vi "Correct_Position_info.vi"() -> (0 "error out":errorcluster, 4 "Path":path)   [LabVIEW 2015]
panel:
  out "File Changed":bool
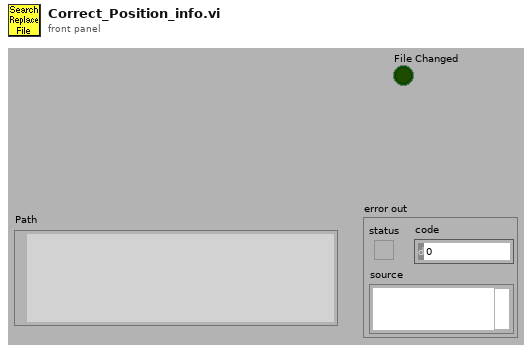
[diagram p1: front panel]
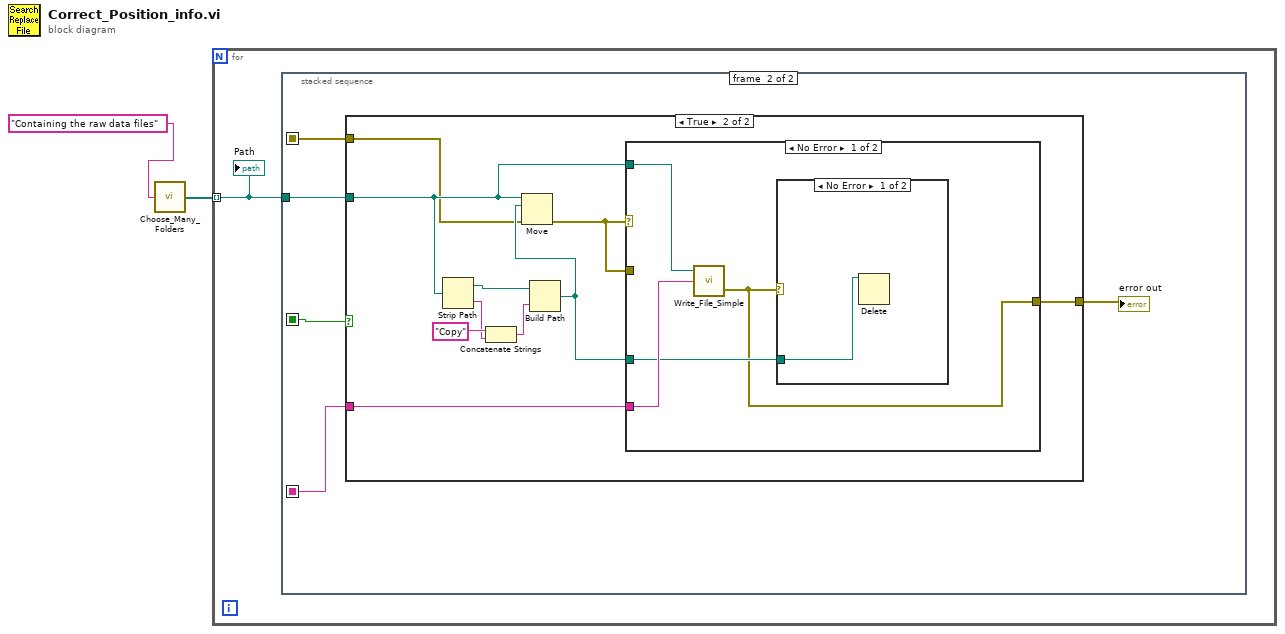
[diagram p0: block diagram]
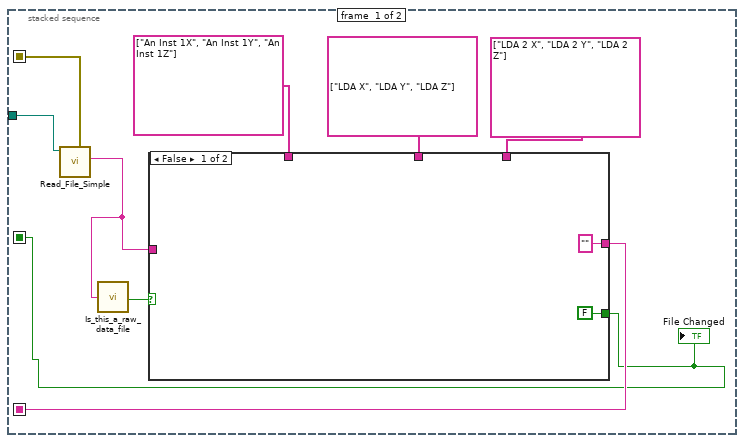
[diagram p2: hidden frame]
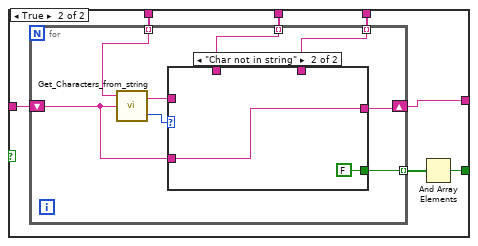
[diagram p3: hidden frame]
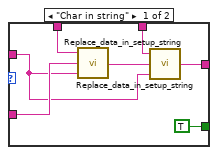
[diagram p4: hidden frame]
diagram:
  n1 = call "Choose_Many_Folders.vi"("Purpose of choosing folder"="Containing the raw data files") -> ("Files"=w1:path[])
  n2 = for {
    tunnel: w1 -> [w3] mode=indexing
    n3 = stacked-sequence {
      seq-local: [w11 _] -> [_ w39]
      seq-local: [w8 _] -> [_ w41]
      seq-local: [w6 _] -> [_ w40]
      tunnel: w3 -> [w12 w43]
      frame #0 {
        n4 = call "Read_File_Simple.vi"("Filename"=w12) -> ("error out"=w11:errorcluster, "string"=w5:string)  [unwired: 4 in, 4 out]
        n5 = call "Is_this_a_raw_data_file.vi"("character string"=w5) -> ("Raw Dat File?"=w4:bool)  [unwired: 2 out]
        n6 = case shown="False" w4 {
          tunnel: string[] ["An Inst 1X", "An Inst 1Y", "An Inst 1Z"] -> [_ w21]
          tunnel: string[] ["LDA X", "LDA Y", "LDA Z"] -> [_ w20]
          tunnel: ["" ("string") w19] -> w8
          tunnel: string[] ["LDA 2 X", "LDA 2 Y", "LDA 2 Z"] -> [_ w18]
          tunnel: [FALSE w16] -> w6
          tunnel: w5 -> [_ w15]
          frame False {
          }
          frame True {
            n7 = for {
              shift-right: [w25] -> w19
              shift-left: w15 -> [w26]
              tunnel: w21 -> [w29] mode=indexing
              tunnel: w20 -> [w28] mode=indexing
              tunnel: w18 -> [w27] mode=indexing
              tunnel: [w22] -> w17 mode=indexing
              n8 = call "Get_Characters_from_string.vi"("Input string"=w26, "Variable name"=w29) -> ("Status"=w23:enum16{"Char in string", "Char not in string"}, "Value"=w24:string)  [unwired: 1 in]
              n9 = case shown="\"Char not in string\"" w23 {
                tunnel: w28 -> [w36 _]
                tunnel: w27 -> [w35 _]
                tunnel: w26 -> [w34 w38]
                tunnel: [w33 w38] -> w25
                tunnel: w24 -> [w31 _]
                tunnel: [TRUE FALSE] -> w22
                frame "Char in string" {
                  n10 = call "Replace_data_in_setup_string.vi"("New data string"=w31, "Input string"=w34, "Variable name"=w36) -> ("Appended string"=w32:string)
                  n11 = call "Replace_data_in_setup_string.vi"("New data string"=w31, "Input string"=w32, "Variable name"=w35) -> ("Appended string"=w33:string)
                }
                frame "Char not in string" {
                }
              }
            }
            n12 = And Array Elements(Boolean array=w17) -> (logical AND=w16:bool)
          }
        }
        "File Changed" <- w6
      }
      frame #1 {
        n13 = case shown="True" w40 {
          tunnel: w43 -> [_ w50]
          tunnel: w41 -> [_ w49]
          tunnel: [w44 w47] -> w42
          tunnel: w39 -> [w44 w45]
          frame False {
          }
          frame True {
            n14 = Strip Path(path=w50) -> (stripped path=w51:path, name=w53:string)
            n15 = Concatenate Strings("Copy" ("name or relative path"), w53) -> (w52:string)
            n16 = Build Path(base path=w51, name or relative path=w52) -> (appended path=w48:path)
            n17 = Move(source path=w50, error in=w45, 10:w48) -> (error out=w46:errorcluster)  [unwired: 2 in, 2 out]
            n18 = case shown="No Error" w46 {
              tunnel: w50 -> [w58 _]
              tunnel: w49 -> [w57 _]
              tunnel: w48 -> [w56 _]
              tunnel: [w55 w60] -> w47
              tunnel: w46 -> [_ w60]
              frame No Error {
                n19 = call "Write_File_Simple.vi"("character string"=w57, "file path"=w58) -> ("error out"=w55:errorcluster)  [unwired: 1 in, 1 out]
                n20 = case shown="No Error" w55 {
                  tunnel: w56 -> [w59 _]
                  frame No Error {
                    n21 = Delete(path (use dialog)=w59) -> ()  [unwired: 4 in, 3 out]
                  }
                  frame Error {
                  }
                }
              }
              frame Error {
              }
            }
          }
        }
        "error out" <- w42
      }
    }
    "Path" <- w3
  }
